vi "Boolean both are true both are false.vi"(10 "Input A":bool, 11 "Input B":bool) -> (2 "output B":bool, 3 "output A":bool)   [LabVIEW 2013]
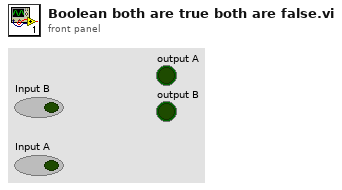
[diagram p1: front panel]
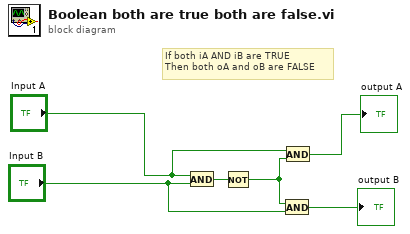
[diagram p0: block diagram]
diagram:
  # "If both iA AND iB are TRUE\nThen both oA and oB are FALSE"
  n1 = And(x="Input A", y="Input B") -> (x .and. y?=w3:bool)
  n2 = Not(x=w3) -> (.not. x?=w4:bool)
  n3 = And(x=w4, y="Input B") -> (x .and. y?=→"output B":bool)
  n4 = And(x="Input A", y=w4) -> (x .and. y?=→"output A":bool)
